vi "Read Compressed Frame (SubVI).vi"(0 "File REF In":refnum<file>) -> (10 "Frame Number":u64, 12 "Stack Number":u64, 14 "File REF Out":refnum<file>, 15 "EOF":bool, 16 "Bit Depth":u8[](array[numeric]), 18 "Minimum":u8[](array[numeric]), 19 "Data":u8[](array[numeric]))   [LabVIEW 2015]
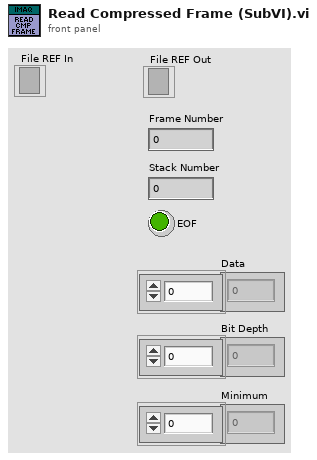
[diagram p1: front panel]
types:
  T1 = enum16{"big-endian, network order", "native, host order", "little-endian"}
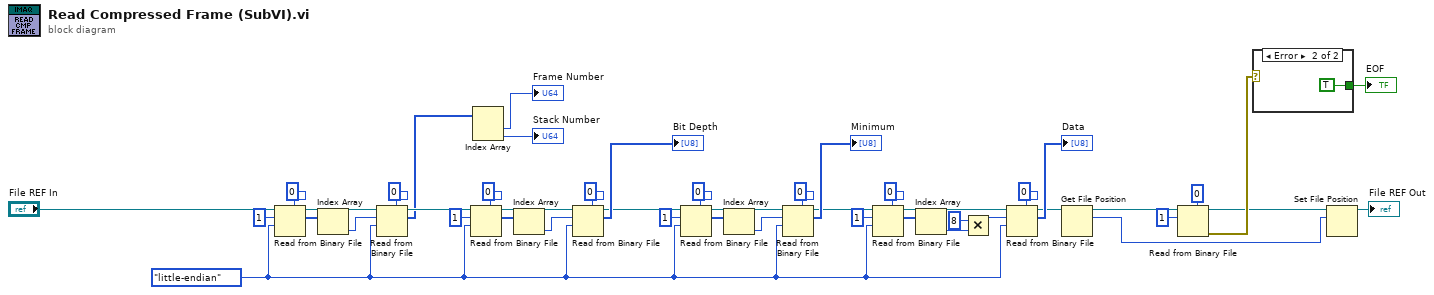
[diagram p0: block diagram]
diagram:
  w43 = T1."little-endian" ("byte order (0:big-endian, network order)")
  n1 = Read from Binary File(5:0 ("count (1)"), 9:w43, 10:1 ("count (1)"), 11:"File REF In") -> (2:w18:i32[], 3:w17:refnum<file>)  [unwired: 2 in, 2 out]
  n2 = Index Array(array=w18) -> (element=w19:i32)  [unwired: 1 in]
  n3 = Read from Binary File(5:u64 0 ("count (1)"), 9:w43, 10:w19, 11:w17) -> (2:w20:u64[], 3:w39:refnum<file>)  [unwired: 2 in, 2 out]
  n4 = Read from Binary File(5:0 ("count (1)"), 9:w43, 10:1 ("count (1)"), 11:w39) -> (2:w22:i32[], 3:w23:refnum<file>)  [unwired: 2 in, 2 out]
  n5 = Index Array(array=w20) -> (element #1=→"Frame Number":u64, element #2=→"Stack Number":u64)  [unwired: 2 in]
  n6 = Index Array(array=w22) -> (element=w21:i32)  [unwired: 1 in]
  n7 = Read from Binary File(5:u8 0 ("count (1)"), 9:w43, 10:w21, 11:w23) -> (2:→"Bit Depth":u8[], 3:w42:refnum<file>)  [unwired: 2 in, 2 out]
  n8 = Read from Binary File(5:0 ("count (1)"), 9:w43, 10:1 ("count (1)"), 11:w42) -> (2:w31:i32[], 3:w30:refnum<file>)  [unwired: 2 in, 2 out]
  n9 = Index Array(array=w31) -> (element=w32:i32)  [unwired: 1 in]
  n10 = Read from Binary File(5:u8 0 ("count (1)"), 9:w43, 10:w32, 11:w30) -> (2:→"Minimum":u8[], 3:w41:refnum<file>)  [unwired: 2 in, 2 out]
  n11 = Read from Binary File(5:0 ("count (1)"), 9:w43, 10:1 ("count (1)"), 11:w41) -> (2:w34:i32[], 3:w35:refnum<file>)  [unwired: 2 in, 2 out]
  n12 = Index Array(array=w34) -> (element=w33:i32)  [unwired: 1 in]
  n13 = Multiply(x=8, y=w33) -> (x*y=w2:i32)
  n14 = Read from Binary File(5:u8 0 ("count (1)"), 9:w43, 10:w2, 11:w35) -> (2:→"Data":u8[], 3:w40:refnum<file>)  [unwired: 2 in, 2 out]
  n15 = Get File Position(7:w40) -> (2:w15:i64, 3:w14:refnum<file>)  [unwired: 1 in, 1 out]
  n16 = Read from Binary File(5:u8 0, 10:1 ("count (1)"), 11:w14) -> (0:w10:errorcluster, 3:w8:refnum<file>)  [unwired: 3 in, 2 out]
  n17 = case shown="Error" w10 {
    tunnel: [_ TRUE] -> w11
    frame No Error {
    }
    frame Error {
    }
  }
  "EOF" <- w11
  n18 = Set File Position(offset (in bytes) (0)=w15, refnum=w8) -> (refnum out=→"File REF Out":refnum<file>)  [unwired: 2 in, 1 out]
